vi "OICB-Set PWM.vi"   [LabVIEW 2015]
uses:
  <vilib>/Rock Robotics/Network Tables/NT Write String.vi
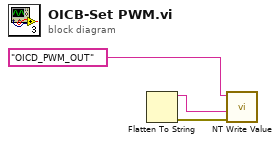
[diagram p0: block diagram]
diagram:
  n1 = Flatten To String() -> (data string=w1:string, error out=w2:errorcluster)  [unwired: 4 in, 1 out]
  n2 = call-poly <vilib>:"NT Write Value.vi"("error in"=w2, "String"=w1, "Name"="OICD_PWM_OUT") -> ()  [unwired: 8 in, 1 out]
